vi "Is Hex.vi"(4 "String":string) -> (7 "Hex":bool)   [LabVIEW 2020, in "URI.lvlib"]
uses:
  URI.lvlib
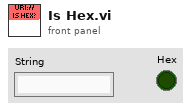
[diagram p1: front panel]
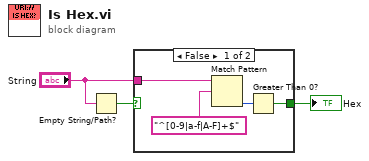
[diagram p0: block diagram]
diagram:
  n1 = Empty String/Path?(string/path="String") -> (empty?=w3:bool)
  n2 = case shown="False" w3 {
    selector: w3 -> [_ w8]
    tunnel: "String" -> [w7 _]
    tunnel: [w4 w8] -> w1
    frame False {
      n3 = Match Pattern(string=w7, regular expression="^[0-9|a-f|A-F]+$") -> (offset past match=w5:i32)  [unwired: 1 in, 3 out]
      n4 = Greater Than 0?(x=w5) -> (x > 0?=w4:bool)
    }
    frame True {
    }
  }
  "Hex" <- w1
